vi "Count Photons.vi"(0 "acquire?":bool, 1 "counter cluster in":T2, 2 "integration cluster in":T1, 3 "pixel counter in":u32, 4 "total pixels acquired in":u64, 5 "photon counts":T4, 6 "TAG slice options":T3, 7 "scan specifications":T5) -> (20 "finished?":bool, 21 "counter cluster out":T2, 22 "integration cluster out":T1, 23 "pixel counter out":u32, 24 "total pixels acquired out":u64)   [LabVIEW 2010]
uses:
  counter_cluster_tagResonant.ctl
  scan_specification_tagResonant.ctl
  integration_cluster.ctl
  common_typedefs/channels_cluster.ctl
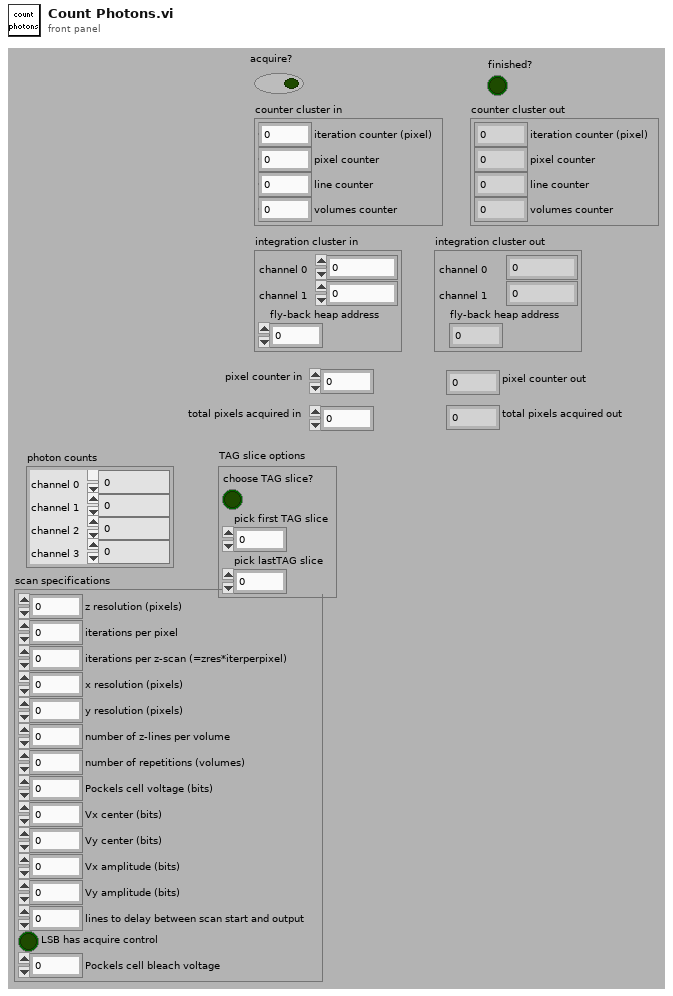
[diagram p1: front panel]
types:
  T1 = typedef "integration_cluster.ctl" = cluster{"channel 0":u32, "channel 1":u32, "fly-back heap address":u32}
  T2 = typedef "counter_cluster_tagResonant.ctl" = cluster{"iteration counter (pixel)":u16, "pixel counter":u16, "line counter":i16, "volumes counter":u16}
  T3 = cluster{"choose TAG slice?":bool, "pick first TAG slice":u32, "pick lastTAG slice":u32}
  T4 = typedef "channels_cluster.ctl" = cluster{"channel 0":u32, "channel 1":u32, "channel 2":u32, "channel 3":u32}
  T5 = typedef "scan_specification_tagResonant.ctl" = cluster{"z resolution (pixels)":u16, "iterations per pixel":u16, "iterations per z-scan (=zres*iterperpixel)":u16, "x resolution (pixels)":u16, "y resolution (pixels)":u16, "number of z-lines per volume":u16, "number of repetitions (volumes)":i32, "Pockels cell voltage (bits)":i16, "Vx center (bits)":i16, "Vy center (bits)":i16, "Vx amplitude (bits)":i16, "Vy amplitude (bits)":i16, "lines to delay between scan start and output":u16, "LSB has acquire control":bool, "Pockels cell bleach voltage":i16}
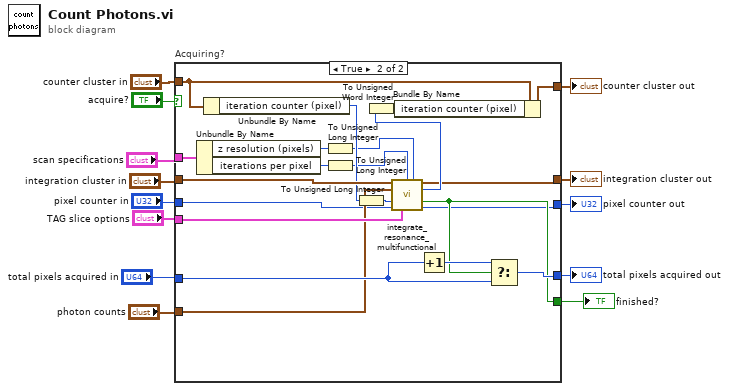
[diagram p0: block diagram]
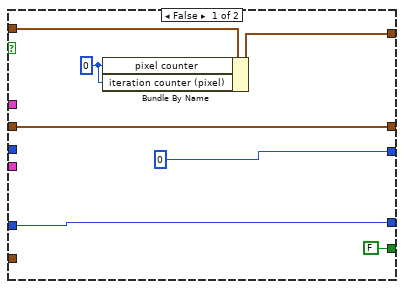
[diagram p2: hidden frame]
diagram:
  n1 = case "Acquiring?" shown="True" "acquire?" {
    tunnel: "counter cluster in" -> [w16 w29]
    tunnel: [w20 w39] -> w4
    tunnel: [w18 w33] -> w3
    tunnel: "integration cluster in" -> [w18 w38]
    tunnel: "photon counts" -> [_ w30]
    tunnel: "total pixels acquired in" -> [w15 w35]
    tunnel: [w15 w37] -> w6
    tunnel: [FALSE ("finished?") w34] -> w5
    tunnel: "TAG slice options" -> [_ w32]
    tunnel: [u32 0 ("pixel counter out") w31] -> w2
    tunnel: "scan specifications" -> [_ w22]
    tunnel: "pixel counter in" -> [_ w21]
    frame False {
      w19 = u16 0 ("pixel counter")
      n2 = Bundle By Name(cluster=w16, "pixel counter"=w19, "iteration counter (pixel)"=w19) -> (w20:T2)
    }
    frame True {
      n3 = Unbundle By Name(w22) -> ("z resolution (pixels)"=w25:u16, "iterations per pixel"=w26:u16)
      n4 = Unbundle By Name(w29) -> ("iteration counter (pixel)"=w28:u16)
      n5 = To Unsigned Long Integer(number=w25) -> (unsigned 32bit integer=w24:u32)
      n6 = To Unsigned Long Integer(number=w26) -> (unsigned 32bit integer=w23:u32)
      n7 = To Unsigned Long Integer(number=w28) -> (unsigned 32bit integer=w27:u32)
      n8 = call "integrate_resonance_multifunctional.vi"("integration cluster in"=w38, "integration iterations per pixel"=w23, "number of pixels"=w24, "sampling values in"=w30, "iteration counter in"=w27, "pixel counter in"=w21, "TAG slice options"=w32) -> ("integration cluster out"=w33:T1, "iteration counter out"=w40:u32, "finished?"=w34:bool, "pixel counter out"=w31:u32)  [unwired: 5 in]
      n9 = To Unsigned Word Integer(number=w40) -> (unsigned 16bit integer=w41:u16)
      n10 = Bundle By Name(cluster=w29, "iteration counter (pixel)"=w41) -> (w39:T2)
      n11 = Increment(x=w35) -> (x+1=w36:u64)
      n12 = Select(t=w36, s=w34, f=w35) -> (s? t:f=w37:u64)
    }
  }
  "total pixels acquired out" <- w6
  "finished?" <- w5
  "counter cluster out" <- w4
  "integration cluster out" <- w3
  "pixel counter out" <- w2
